vi "Begin.vi"(11 "Image Size":T1=enum."160x120") -> (0 "error out":errorcluster)   [LabVIEW 2011]
doc: "Called before other user functions, this VI is expected to open initial I/O refnums, load in file data, and do all program initialization. Notice that the <B>error out</B> terminal is simply used for data flow. Wiring it to other structures or subVIs ensures that this VI runs first."
uses:
  <vilib>/Rock Robotics/WPI/Camera/WPI_CameraImageSize.ctl
  <vilib>/Rock Robotics/SystemInterfaces/DIO/FPGA_DIOPWMChannel.ctl
  <vilib>/Rock Robotics/WPI/Joystick/WPI_JoystickDeviceEnum.ctl
  <vilib>/Rock Robotics/SystemInterfaces/DIO/FPGA_DIOChannel.ctl
  <vilib>/Rock Robotics/SystemInterfaces/AI/FPGA_AIGyroChannel.ctl
  <vilib>/Rock Robotics/WPI/Camera/WPI_CameraWhite Balance Values.ctl
  <vilib>/Rock Robotics/WPI/Camera/WPI_CameraExposure Values.ctl
  <vilib>/Rock Robotics/WPI/Camera/WPI_CameraFrameRate.ctl
  <vilib>/Rock Robotics/WPI/MotorControl/WPI_MotorControlOpen Victor.vi
  Robot Global Data.vi
  <vilib>/Rock Robotics/SystemInterfaces/Typedef/FPGA_TypedefDigitalModule.ctl
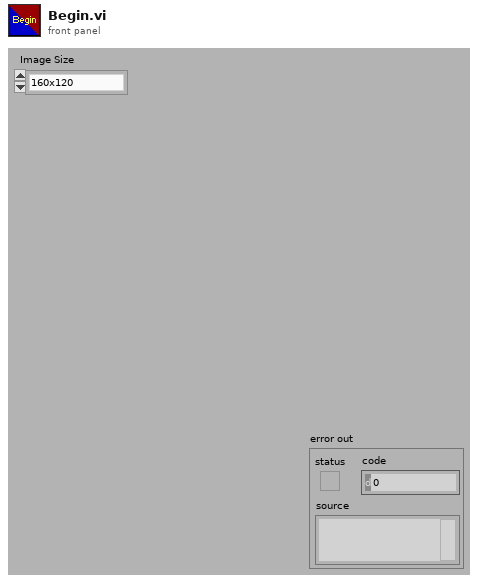
[diagram p1: front panel]
types:
  T1 = typedef "WPI_CameraImageSize.ctl" = enum16{"640x480", "320x240", "160x120"}
  T2 = typedef "WPI_CameraFrameRate.ctl" = u32
  T3 = typedef "WPI_CameraExposure Values.ctl" = enum16{"Auto", "Flicker-free 50 Hz", "Flicker-free 60 Hz", "Hold current"}
  T4 = typedef "WPI_CameraWhite Balance Values.ctl" = enum16{"Auto", "Fixed indoor", "Fixed outdoor 1", "Fixed outdoor 2", "Fixed fluorescent 1", "Fixed fluorescent 2", "Hold current"}
  T5 = typedef "FPGA_DIOPWMChannel.ctl" = enum8{"PWM 1", "PWM 2", "PWM 3", "PWM 4", "PWM 5", "PWM 6", "PWM 7", "PWM 8", "PWM 9", "PWM 10", "Invalid"}
  T6 = typedef "FPGA_AIGyroChannel.ctl" = enum8{"AI 1", "AI 2", "Invalid"}
  T7 = typedef "FPGA_DIOChannel.ctl" = enum8{"DIO 1", "DIO 2", "DIO 3", "DIO 4", "DIO 5", "DIO 6", "DIO 7", "DIO 8", "DIO 9", "DIO 10", "DIO 11", "DIO 12", "DIO 13", "DIO 14", "Invalid"}
  T8 = typedef "WPI_JoystickDeviceEnum.ctl" = enum16{"USB 1", "USB 2", "USB 3", "USB 4", "Kinect 1", "Kinect 2"}
  T9 = typedef "FPGA_TypedefDigitalModule.ctl" = enum16{"Digital Module 1", "Digital Module 2"}
  T10 = typedef "WPI_I2CDevRef.ctl" = cluster{"DevStatus":errorcluster, "Digital Module":T9, "Device Address":u8}
  T11 = typedef "WPI_MotorControlDeviceRef.ctl" = cluster{"DeviceStatus":errorcluster, "Type":enum16{"PWM", "CAN"}, "PWM":cluster{"Digital Module":T9, "PWM Channel":T5, "DeadBand":T12}, "CAN":cluster{"Device Number":u8, "Control Mode":T13, "Semaphore":T14, "Max Vout":dbl}, "Invert":bool, "TransformRef":T15, "InvTransformRef":T15}
  T12 = typedef "WPI_PWMDeadband.ctl" = cluster{"Name":string, "maxPositivePwm":i32, "minPositivePwm":i32, "centerPwm":i32, "maxNegativePwm":i32, "minNegativePwm":i32, "angularRange":u16}
  T13 = typedef "WPI_CANJaguar_ControlMode.ctl" = enum8{"Percent VBus", "Current", "Speed", "Position", "Voltage"}
  T14 = typedef "Semaphore RefNum" = refnum<k1>
  T15 = typedef "WPI_PWMTransform_ConPane.ctl" = refnum<vi>
  T16 = typedef "WPI_CameraDevRef.ctl" = cluster{"Camera Address":string, "CameraStatus":errorcluster, "Acquire Image Notifier":refnum<notifier>}
  T17 = typedef "WPI_JoystickDevRef.ctl" = cluster{"Device":T8}
  T18 = typedef "WPI_ServoDeviceRef.ctl" = cluster{"DeviceStatus":errorcluster, "Digital Module":T9, "PWM Channel":T5, "DeadBand":T12}
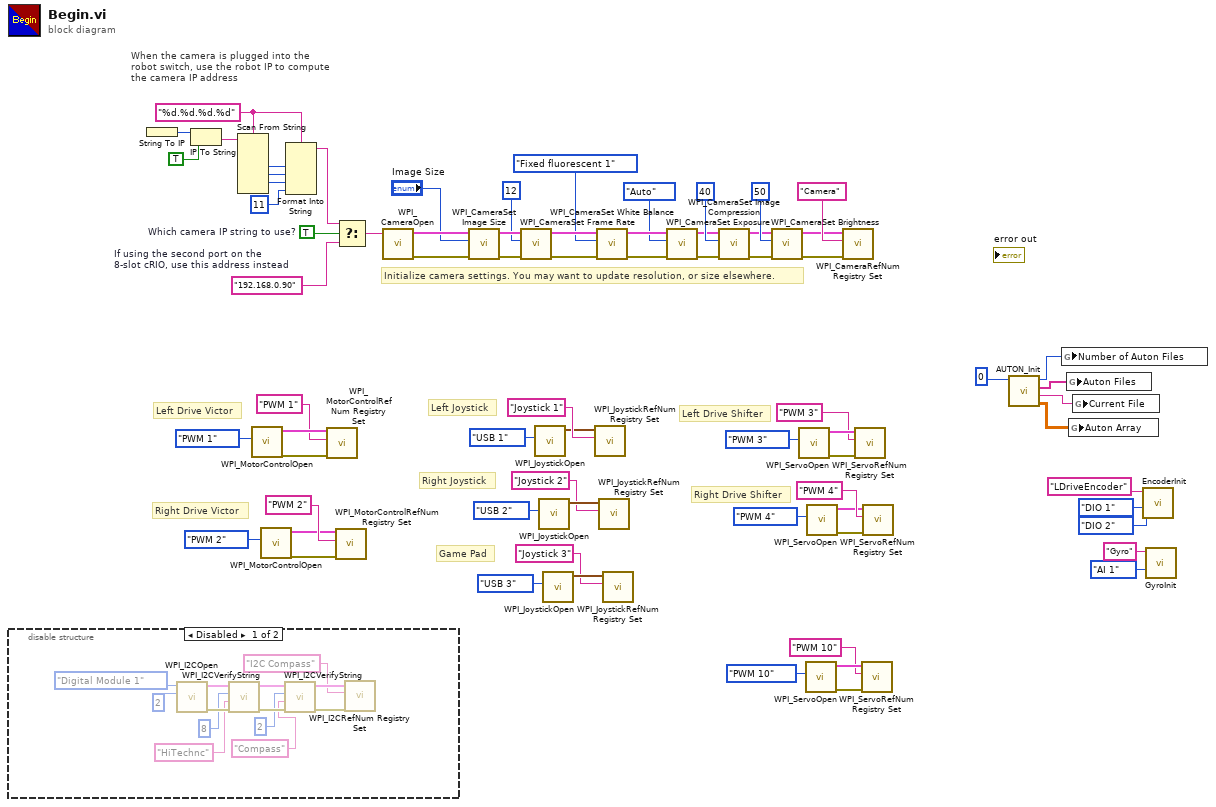
[diagram p0: block diagram]
diagram:
  w1 = TRUE  # Which camera IP string to use?
  w5 = "%d.%d.%d.%d" ("format string")
  w2 = "192.168.0.90"  # If using the second port on the 8-slot cRIO, use this address instead
  # "When the camera is plugged into the\nrobot switch, use the robot IP to compute\nthe camera IP address"
  # "Initialize camera settings. You may want to update resolution, or size elsewhere."
  # "Right Drive Shifter"
  # "Left Drive Shifter"
  # "Right Joystick"
  # "Left Joystick"
  # "Game Pad"
  # "Right Drive Victor"
  # "Left Drive Victor"
  n1 = disable-structure shown="Disabled" {
    frame Disabled {
      n2 = call <vilib>:"WPI_I2COpen.vi"("Device Address"=u8 2, "Digital Module (Module 1)"=FPGA_TypedefDigitalModule."Digital Module 1") -> ("error out"=w85:errorcluster, "I2CDevRef"=w84:T10)  [unwired: 8 in]
      n3 = call <vilib>:"WPI_I2CVerifyString.vi"("error in (no error)"=w85, "Expected"="HiTechnc", "Register Address"=u8 8, "I2CDevRef"=w84) -> ("error out"=w83:errorcluster, "I2CDevRef"=w82:T10)  [unwired: 6 in]
      n4 = call <vilib>:"WPI_I2CVerifyString.vi"("error in (no error)"=w83, "Expected"="Compass", "Register Address"=u8 2, "I2CDevRef"=w82) -> ("error out"=w81:errorcluster, "I2CDevRef"=w80:T10)  [unwired: 6 in]
      n5 = call <vilib>:"WPI_I2CRefNum Registry Set.vi"("error in (no error)"=w81, "refnum name"="I2C Compass", "I2CDevRef"=w80) -> ()  [unwired: 7 in, 2 out]
    }
    frame Enabled {
    }
  }
  n6 = String To IP() -> (0:w12:u32)  [unwired: 1 in]
  n7 = IP To String(1:TRUE ("dot notation? (F)"), 2:w12) -> (0:w10:string)
  n8 = Scan From String(format string=w5, input string=w10) -> (output 1=w9:i32, output 2=w8:i32, output 3=w7:i32)  [unwired: 7 in, 3 out]
  n9 = call-poly <vilib>:"WPI_MotorControlOpen.vi"("PWM Channel"=FPGA_DIOPWMChannel."PWM 1") -> ("error out"=w71:errorcluster, "MotorControlDeviceRef"=w72:T11)  [unwired: 9 in]
  n10 = call-poly <vilib>:"WPI_MotorControlOpen.vi"("PWM Channel"=FPGA_DIOPWMChannel."PWM 2") -> ("error out"=w66:errorcluster, "MotorControlDeviceRef"=w65:T11)  [unwired: 9 in]
  n11 = Format Into String(format string=w5, w9, w8, w7, 11 ("Compression")) -> (resulting string=w3:string)  [unwired: 2 in, 1 out]
  n12 = call <vilib>:"WPI_MotorControlRefNum Registry Set.vi"("error in (no error)"=w71, "refnum name"="PWM 1", "MotorControlDevRef"=w72) -> ()  [unwired: 7 in, 2 out]
  n13 = call <vilib>:"WPI_MotorControlRefNum Registry Set.vi"("error in (no error)"=w66, "refnum name"="PWM 2", "MotorControlDevRef"=w65) -> ()  [unwired: 7 in, 2 out]
  n14 = Select(t=w3, s=w1, f=w2) -> (s? t:f=w4:string)
  n15 = call <vilib>:"WPI_CameraOpen.vi"("Camera Address"=w4) -> ("error out"=w24:errorcluster, "CameraDevRef"=w25:T16)  [unwired: 1 in, 8 out]
  n16 = call <vilib>:"WPI_CameraSet Image Size.vi"("error in (no error)"=w24, "Image Size"="Image Size", "CameraDevRef"=w25) -> ("error out"=w23:errorcluster, "CameraDevRef Out"=w26:T16)  [unwired: 7 out]
  n17 = call <vilib>:"WPI_CameraSet Frame Rate.vi"("error in (no error)"=w23, "Frame Rate (fps)"=T2 12, "CameraDevRef"=w26) -> ("error out"=w22:errorcluster, "CameraDevRef Out"=w28:T16)  [unwired: 7 out]
  n18 = call <vilib>:"WPI_JoystickOpen.vi"("JoystickDevice"=WPI_JoystickDeviceEnum."USB 1") -> ("JoystickDevRef"=w56:T17)  [unwired: 10 in]
  n19 = call <vilib>:"WPI_JoystickOpen.vi"("JoystickDevice"=WPI_JoystickDeviceEnum."USB 2") -> ("JoystickDevRef"=w61:T17)  [unwired: 10 in]
  n20 = call <vilib>:"WPI_JoystickOpen.vi"("JoystickDevice"=WPI_JoystickDeviceEnum."USB 3") -> ("JoystickDevRef"=w64:T17)  [unwired: 10 in]
  n21 = call <vilib>:"WPI_JoystickRefNum Registry Set.vi"("refnum name"="Joystick 1", "JoystickDevRef"=w56) -> ()  [unwired: 8 in, 2 out]
  n22 = call <vilib>:"WPI_CameraSet White Balance.vi"("error in (no error)"=w22, "White Balance"=WPI_CameraWhite_Balance_Values."Fixed fluorescent 1", "CameraDevRef"=w28) -> ("error out"=w21:errorcluster, "CameraDevRef Out"=w27:T16)  [unwired: 7 out]
  n23 = call <vilib>:"WPI_JoystickRefNum Registry Set.vi"("refnum name"="Joystick 2", "JoystickDevRef"=w61) -> ()  [unwired: 8 in, 2 out]
  n24 = call <vilib>:"WPI_JoystickRefNum Registry Set.vi"("refnum name"="Joystick 3", "JoystickDevRef"=w64) -> ()  [unwired: 8 in, 2 out]
  n25 = call <vilib>:"WPI_CameraSet Exposure.vi"("error in (no error)"=w21, "Exposure"=WPI_CameraExposure_Values."Auto", "CameraDevRef"=w27) -> ("error out"=w20:errorcluster, "CameraDevRef Out"=w30:T16)  [unwired: 7 out]
  n26 = call <vilib>:"WPI_CameraSet Image Compression.vi"("error in (no error)"=w20, "Compression"=40, "CameraDevRef"=w30) -> ("error out"=w19:errorcluster, "CameraDevRef Out"=w29:T16)  [unwired: 7 out]
  n27 = call <vilib>:"WPI_CameraSet Brightness.vi"("error in (no error)"=w19, "Brightness"=50, "CameraDevRef"=w29) -> ("error out"=w17:errorcluster, "CameraDevRef Out"=w18:T16)  [unwired: 7 out]
  n28 = call <vilib>:"WPI_ServoOpen.vi"("PWM Channel"=FPGA_DIOPWMChannel."PWM 3") -> ("error out"=w55:errorcluster, "ServoDeviceRef"=w54:T18)  [unwired: 9 in]
  n29 = call <vilib>:"WPI_ServoOpen.vi"("PWM Channel"=FPGA_DIOPWMChannel."PWM 10") -> ("error out"=w37:errorcluster, "ServoDeviceRef"=w36:T18)  [unwired: 9 in]
  n30 = call <vilib>:"WPI_ServoOpen.vi"("PWM Channel"=FPGA_DIOPWMChannel."PWM 4") -> ("error out"=w48:errorcluster, "ServoDeviceRef"=w49:T18)  [unwired: 9 in]
  n31 = call <vilib>:"WPI_CameraRefNum Registry Set.vi"("error in (no error)"=w17, "refnum name"="Camera", "CameraDevRef"=w18) -> ()  [unwired: 9 out]
  n32 = call <vilib>:"WPI_ServoRefNum Registry Set.vi"("error in (no error)"=w55, "refnum name"="PWM 3", "ServoDeviceRef"=w54) -> ()  [unwired: 7 in, 2 out]
  n33 = call <vilib>:"WPI_ServoRefNum Registry Set.vi"("error in (no error)"=w37, "refnum name"="PWM 10", "ServoDeviceRef"=w36) -> ()  [unwired: 7 in, 2 out]
  n34 = call <vilib>:"WPI_ServoRefNum Registry Set.vi"("error in (no error)"=w48, "refnum name"="PWM 4", "ServoDeviceRef"=w49) -> ()  [unwired: 7 in, 2 out]
  n35 = call "AUTON_Init.vi"("Default File"=0) -> ("Auton Array"=w45:dbl[][], "Current File"=w44:string, "Auton Files"=w46:string[], "Number of Auton Files"=w47:i64)  [unwired: 7 in]
  n36 = global write "Robot Global Data.vi" "Number of Auton Files"(w47) -> ()
  n37 = global write "Robot Global Data.vi" "Auton Files"(w46) -> ()
  n38 = global write "Robot Global Data.vi" "Auton Array"(w45) -> ()
  n39 = global write "Robot Global Data.vi" "Current File"(w44) -> ()
  n40 = call "EncoderInit.vi"("refnum name"="LDriveEncoder", "DIO Channel"=FPGA_DIOChannel."DIO 1", "DIO Channel 2"=FPGA_DIOChannel."DIO 2") -> ()  [unwired: 8 in]
  n41 = call "GyroInit.vi"("refnum name"="Gyro", "Analog Channel"=FPGA_AIGyroChannel."AI 1") -> ()  [unwired: 8 in]
